vi "TTA_MATLAB_RFIC_RX_Enable.vi"(0 "Channels":string[](array[combo]), 11 "error in":errorcluster) -> (4 "SuccessComm":bool[](array[boolean]), 15 "error out":errorcluster)   [LabVIEW 2016]
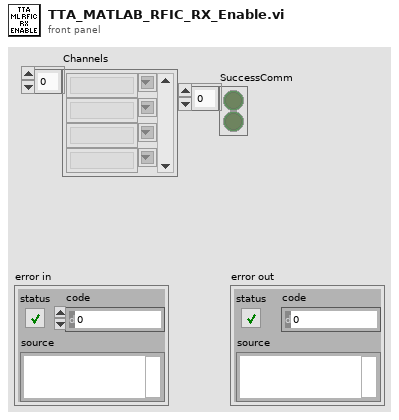
[diagram p1: front panel]
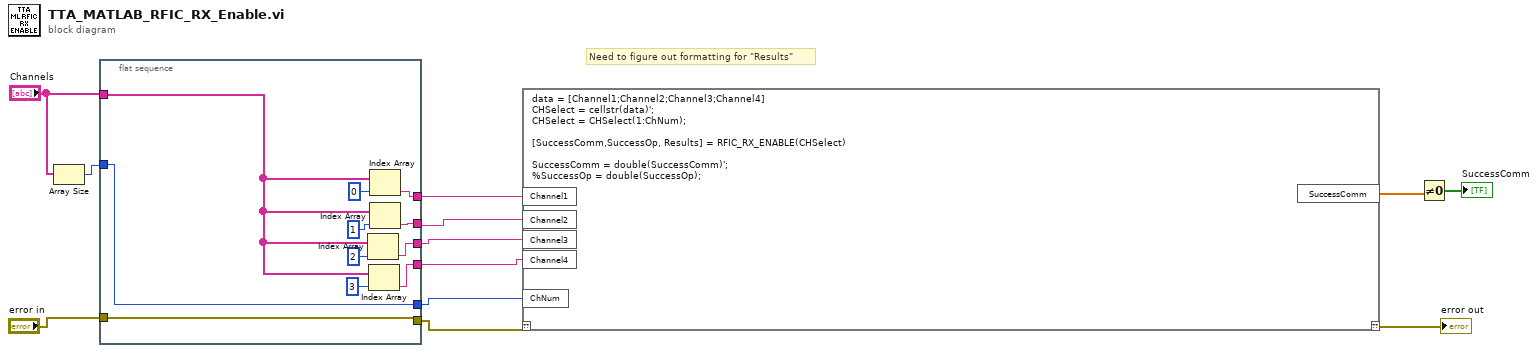
[diagram p0: block diagram]
diagram:
  # "Need to figure out formatting for \"Results\""
  n1 = Array Size(array="Channels") -> (size(s)=w8:i32)
  n2 = flat-sequence {
    tunnel: "error in" -> [w23]
    tunnel: [w22] -> w7
    tunnel: w8 -> [w16]
    tunnel: [w23] -> w6
    tunnel: "Channels" -> [w15]
    tunnel: [w19] -> w4
    tunnel: [w17] -> w3
    tunnel: [w16] -> w1
    tunnel: [w13] -> w2
    frame #0 {
      n3 = Index Array(array=w15, index=2) -> (element=w17:string)
      n4 = Index Array(array=w15, index=3) -> (element=w13:string)
      n5 = Index Array(array=w15, index=0) -> (element=w22:string)
      n6 = Index Array(array=w15, index=1) -> (element=w19:string)
    }
  }
  n7 = script code="data = [Channel1;Channel2;Channel3;Channel4]\nCHSelect = cellstr(data)';\nCHSelect = CHSelect(1:ChNum);\n\n[SuccessComm,SuccessOp, Results] = RFIC_RX_ENABLE(CHSelect)\n\nSuccessComm = double(SuccessComm)';\n%SuccessOp = double(SuccessOp);"("??"=w6, "Channel1"=w7, "ChNum"=w1, "Channel2"=w4, "Channel3"=w3, "Channel4"=w2) -> ("??"=→"error out":errorcluster, "SuccessComm"=w10:dbl[])
  n8 = Not Equal To 0?(x=w10) -> (x != 0?=→"SuccessComm":bool[])
